vi "cmd1.vi"(6 "Param":string) -> (0 "error out":errorcluster, 2 "reversed":string)   [LabVIEW 2010]
doc: "just testing"
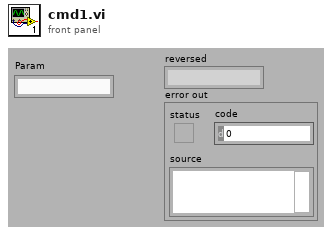
[diagram p1: front panel]
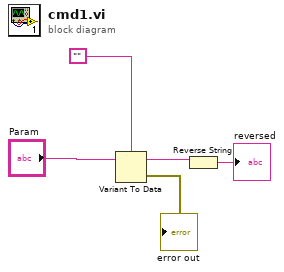
[diagram p0: block diagram]
diagram:
  n1 = Variant To Data(Variant="Param", type="") -> (error out=→"error out":errorcluster, data=w3:string)  [unwired: 1 in]
  n2 = Reverse String(1:w3) -> (0:→"reversed":string)
